vi "ArduinoGrab.vi"(8 "error in (no error)":errorcluster, 11 "DataCluster":T1) -> (0 "error out":errorcluster, 1 "Bytes at Port":u32, 2 "read buffer out":string, 3 "DataCluster out":T1)   [LabVIEW 2020]
uses:
  DataCluster.ctl
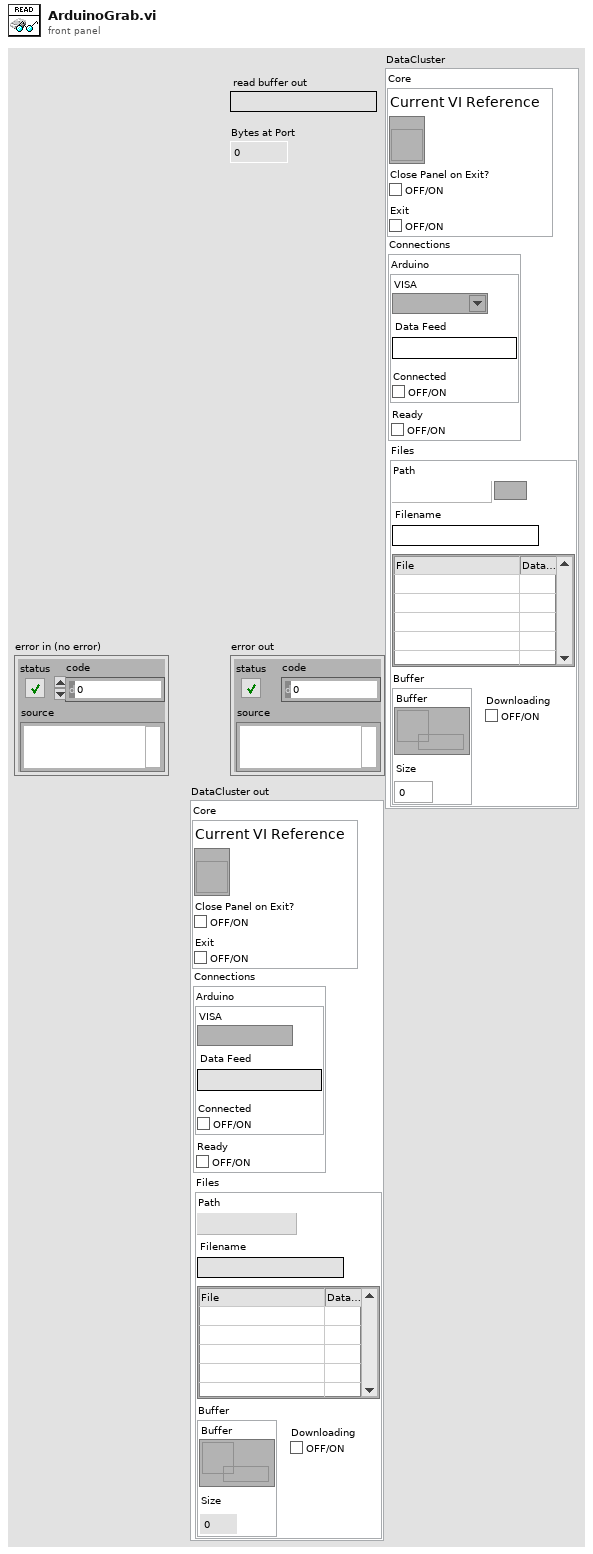
[diagram p1: front panel]
types:
  T1 = typedef "DataCluster.ctl" = cluster{"Core":cluster{"Current VI Reference":refnum<vi>, "Close Panel on Exit?":bool, "Exit":bool}, "Connections":cluster{"Arduino":cluster{"VISA":refnum<visa-resource-name>, "Data Feed":string, "Connected":bool}, "Ready":bool}, "Files":cluster{"Path":path, "Filename":string, "File List":i32, "Buffer":cluster{"Buffer":refnum<queue>, "Size":i32}, "Downloading":bool}}
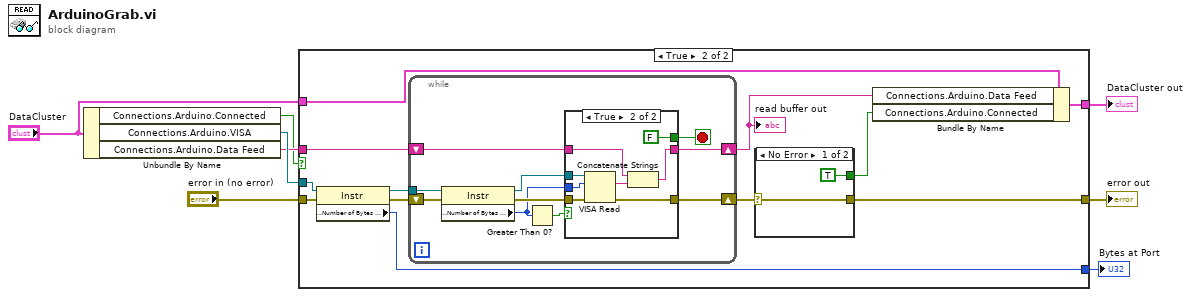
[diagram p0: block diagram]
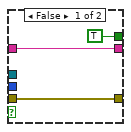
[diagram p3: hidden frame]
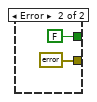
[diagram p4: hidden frame]
diagram:
  n1 = Unbundle By Name("DataCluster") -> ("Connections.Arduino.Connected"=w3:bool, "Connections.Arduino.VISA"=w7:refnum<visa-resource-name>, "Connections.Arduino.Data Feed"=w6:string)
  n2 = case shown="True" w3 {
    tunnel: "error in (no error)" -> [w9 w14]
    tunnel: w7 -> [_ w15]
    tunnel: w6 -> [_ w22]
    tunnel: "DataCluster" -> [w10 w21]
    tunnel: [w10 w19] -> w4
    tunnel: [w9 w17] -> w2
    tunnel: [_ w11] -> w1
    frame False {
    }
    frame True {
      n3 = property class="Instr"(reference=w15, error in=w14) -> (reference out=w12:refnum<visa-resource-name>, error out=w13:errorcluster, "Serial Settings:Number of Bytes at Serial Port"=w11:u32)
      n4 = while {
        tunnel: w12 -> [w31]
        shift-right: [w24] -> w18
        shift-left: w13 -> [w32]
        shift-right: [w25] -> w20
        shift-left: w22 -> [w26]
        stop <- w23 stop-if-true
        n5 = property class="Instr"(reference=w31, error in=w32) -> (reference out=w30:refnum<visa-resource-name>, error out=w29:errorcluster, "Serial Settings:Number of Bytes at Serial Port"=w27:u32)
        n6 = Greater Than 0?(x=w27) -> (x > 0?=w28:bool)
        n7 = case shown="True" w28 {
          tunnel: w30 -> [_ w43]
          tunnel: w29 -> [w35 w42]
          tunnel: [w35 w41] -> w24
          tunnel: w27 -> [_ w40]
          tunnel: [w34 w37] -> w25
          tunnel: w26 -> [w34 w38]
          tunnel: [TRUE FALSE] -> w23
          frame False {
          }
          frame True {
            n8 = VISA Read(VISA resource name=w43, byte count=w40, error in (no error)=w42) -> (read buffer=w39:string, error out=w41:errorcluster)  [unwired: 2 out]
            n9 = Concatenate Strings(w38, w39) -> (w37:string)
          }
        }
      }
      "read buffer out" <- w20
      n10 = case shown="No Error" w18 {
        selector: w18 -> [w45 _]
        tunnel: [w45 errorcluster {"status"=FALSE, "code"=0, "source"=""} ("error IO")] -> w17
        tunnel: [TRUE FALSE] -> w16
        frame No Error {
        }
        frame Error {
        }
      }
      n11 = Bundle By Name(cluster=w21, "Connections.Arduino.Data Feed"=w20, "Connections.Arduino.Connected"=w16) -> (w19:T1)
    }
  }
  "DataCluster out" <- w4
  "error out" <- w2
  "Bytes at Port" <- w1
